vi "Build Target Table.vi"(9 "Search":refnum<class "Search.lvclass">, 10 "Targets In":refnum<vi>[](array[refnum]), 11 "Scope":T1) -> (2 "Targets":refnum<vi>[](array[refnum]), 3 "Target Table":string[][](array[string]))   [LabVIEW 2016, in "Better Search.lvlib" / "BetterSearch.lvclass"]
uses:
  BetterSearch.lvclass
  Search/Search.lvclass
  Data Types/Search Scope.ctl
  Better Search.lvlib
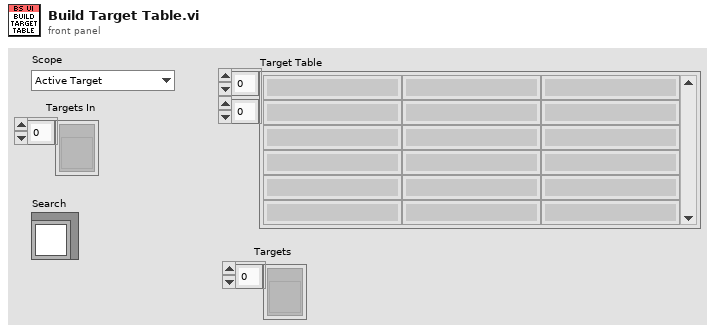
[diagram p1: front panel]
types:
  T1 = typedef "Better Search.lvlib/Search Scope.ctl" = enum16{"Active Target", "Active Project", "Specific Targets", "Active VI", "Active Hierarchy"}
  T2 = typedef "Better Search.lvlib/Search Context.ctl" = cluster{"Type ID":string, "VI Refnum":refnum<vi>, "Starting Text":string, "Shift?":bool, "App Ref":refnum<vi>, "Start Search Type":T3, "Item Graph":T4[], "Variant":variant}
  T3 = typedef "Better Search.lvlib/Start Search Type.ctl" = enum16{"Auto", "Text", "Data Type", "Bundle"}
  T4 = typedef "Better Search.lvlib/Type Reflection Item.ctl" = cluster{"Parent":i32, "Depth":i32, "Children":i32[], "Skip":bool, "Name":string, "Type":variant, "TypeID":string}
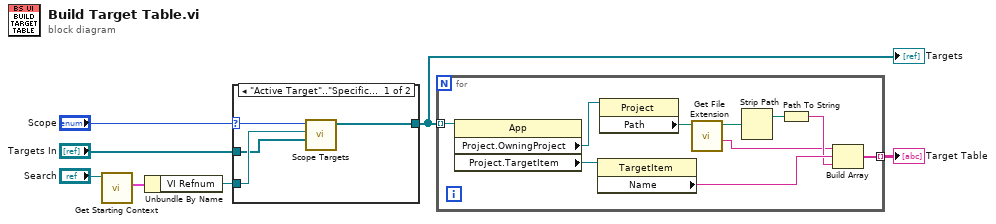
[diagram p0: block diagram]
diagram:
  n1 = call "Get Starting Context.vi"("Search in"="Search") -> ("Starting Context"=w7:T2)  [unwired: 8 in, 2 out]
  n2 = Unbundle By Name(w7) -> ("VI Refnum"=w6:refnum<vi>)
  n3 = case shown="\"Active Target\"..\"Specific Targets\"" "Scope" {
    selector: "Scope" -> [w11 _]
    tunnel: "Targets In" -> [w9 _]
    tunnel: w6 -> [w10 _]
    tunnel: [w8 _] -> w1
    frame "Active Target".."Specific Targets" {
      n4 = call "Scope Targets.vi"("Specific Targets"=w9, "Launching VI"=w10, "Search Scope"=w11) -> ("Scope Targets"=w8:refnum<vi>[])  [unwired: 8 in]
    }
    frame "Active VI", "Active Hierarchy" {
    }
  }
  "Targets" <- w1
  n5 = for {
    tunnel: w1 -> [w21] mode=indexing
    tunnel: [w15] -> w2 mode=indexing
    n6 = property class="App"(reference=w21) -> ("Project.OwningProject"=w20:refnum<vi>, "Project.TargetItem"=w19:refnum<vi>)  [unwired: 1 in, 2 out]
    n7 = property class="TargetItem"(reference=w19) -> ("Name"=w17:string)  [unwired: 1 in, 2 out]
    n8 = property class="Project"(reference=w20) -> ("Path"=w14:path)  [unwired: 1 in, 2 out]
    n9 = call <vilib>:"Get File Extension.vi"("file"=w14) -> ("filename without extension"=w12:string, "dup file"=w13:path)  [unwired: 6 in, 3 out]
    n10 = Strip Path(path=w13) -> (stripped path=w18:path)  [unwired: 1 out]
    n11 = Path To String(path=w18) -> (string=w16:string)
    n12 = Build Array(w12, w17, w16) -> (w15:string[])
  }
  "Target Table" <- w2
